vi "Fitting to battery model.vi"() -> ()   [LabVIEW 2013]
uses:
  <vilib>/Analysis/6fits.llb/Curve Fitting Criteria.ctl
  <vilib>/gmath/NumericalOptimization/Nonlinear Curve Fit LM bound.vi
  <vilib>/gmath/NI_Gmath.lvlib
  <vilib>/Analysis/NI_AALPro.lvlib
panel:
  out "residue":dbl
  out "number of function calls":i32
  out "Nyquist":cluster{dbl[], dbl[]}[](graph)
  out "p_best":dbl[](array[numeric])
  in  "p_init":dbl[](array[numeric])=[1e-06, 0.1, 0.1, 100.0, 1.0, 0.1, 0.1, 10.0, 0.1]
  out "f":dbl[](array[numeric])
  out "z":cdb[](array[numeric])
  in  "String":string="         1.000000E+4\t         4.126488E-2\t         2.967524E-1\n         8.912509E+3\t         4.158981E-2\t         2.604928E-1\n         7.943282E+3\t         4.199738E-2\t         2.277047E-1\n         7.079458E+3\t         4.250813E-2\t         1.979590E-1\n         6.309573E+3\t         4.314743E-2\t         1.708694E-1\n         5.623413E+3\t         4.394647E-2\t         1.460881E-1\n         5.011872E+3\t         4.494331E-2\t         1.233026E-1\n         4.466836E+3\t         4.618408E-2\t         1.022327E-1\n         3.981072E+3\t         4.772409E-2\t         8.262973E-2\n         3.548134E+3\t         4.962877E-2\t         6.427518E-2\n         3.162278E+3\t         5.197420E-2\t         4.698188E-2\n         2.818383E+3\t         5.484690E-2\t         3.059545E-2\n         2.511886E+3\t         5.834239E-2\t         1.499719E-2\n         2.238721E+3\t         6.256184E-2\t         1.075807E-4\n         1.995262E+3\t         6.760643E-2\t        -1.410996E-2\n         1.778279E+3\t         7.356869E-2\t        -2.764623E-2\n         1.584893E+3\t         8.052083E-2\t        -4.044574E-2\n         1.412538E+3\t         8.850068E-2\t        -5.241030E-2\n         1.258925E+3\t         9.749691E-2\t        -6.340858E-2\n         1.122018E+3\t         1.074364E-1\t        -7.329263E-2\n         1.000000E+3\t         1.181775E-1\t        -8.192073E-2\n         8.912509E+2\t         1.295128E-1\t        -8.918393E-2\n         7.943282E+2\t         1.411830E-1\t        -9.503155E-2\n         7.079458E+2\t         1.529012E-1\t        -9.948971E-2\n         6.309573E+2\t         1.643841E-1\t        -1.026685E-1\n         5.623413E+2\t         1.753820E-1\t        -1.047558E-1\n         5.011872E+2\t         1.857037E-1\t        -1.059995E-1\n         4.466836E+2\t         1.952307E-1\t        -1.066836E-1\n         3.981072E+2\t         2.039205E-1\t        -1.071023E-1\n         3.548134E+2\t         2.118007E-1\t        -1.075386E-1\n         3.162278E+2\t         2.189580E-1\t        -1.082484E-1\n         2.818383E+2\t         2.255252E-1\t        -1.094519E-1\n         2.511886E+2\t         2.316687E-1\t        -1.113294E-1\n         2.238721E+2\t         2.375799E-1\t        -1.140211E-1\n         1.995262E+2\t         2.434684E-1\t        -1.176284E-1\n         1.778279E+2\t         2.495579E-1\t        -1.222139E-1\n         1.584893E+2\t         2.560848E-1\t        -1.278009E-1\n         1.412538E+2\t         2.632954E-1\t        -1.343701E-1\n         1.258925E+2\t         2.714434E-1\t        -1.418538E-1\n         1.122018E+2\t         2.807835E-1\t        -1.501279E-1\n         1.000000E+2\t         2.915610E-1\t        -1.590041E-1\n         8.912509E+1\t         3.039956E-1\t        -1.682222E-1\n         7.943282E+1\t         3.182595E-1\t        -1.774476E-1\n         7.079458E+1\t         3.344495E-1\t        -1.862767E-1\n         6.309573E+1\t         3.525587E-1\t        -1.942534E-1\n         5.623413E+1\t         3.724514E-1\t        -2.009005E-1\n         5.011872E+1\t         3.938493E-1\t        -2.057633E-1\n         4.466836E+1\t         4.163370E-1\t        -2.084605E-1\n         3.981072E+1\t         4.393888E-1\t        -2.087338E-1\n         3.548134E+1\t         4.624172E-1\t        -2.064840E-1\n         3.162278E+1\t         4.848327E-1\t        -2.017841E-1\n         2.818383E+1\t         5.061048E-1\t        -1.948662E-1\n         2.511886E+1\t         5.258096E-1\t        -1.860854E-1\n         2.238721E+1\t         5.436572E-1\t        -1.758711E-1\n         1.995262E+1\t         5.594965E-1\t        -1.646750E-1\n         1.778279E+1\t         5.733007E-1\t        -1.529281E-1\n         1.584893E+1\t         5.851424E-1\t        -1.410095E-1\n         1.412538E+1\t         5.951632E-1\t        -1.292303E-1\n         1.258925E+1\t         6.035461E-1\t        -1.178289E-1\n         1.122018E+1\t         6.104913E-1\t        -1.069753E-1\n         1.000000E+1\t         6.161994E-1\t        -9.677938E-2\n         8.912509E+0\t         6.208601E-1\t        -8.730281E-2\n         7.943282E+0\t         6.246451E-1\t        -7.856953E-2\n         7.079458E+0\t         6.277055E-1\t        -7.057593E-2\n         6.309573E+0\t         6.301713E-1\t        -6.329917E-2\n         5.623413E+0\t         6.321524E-1\t        -5.670382E-2\n         5.011872E+0\t         6.337403E-1\t        -5.074691E-2\n         4.466836E+0\t         6.350109E-1\t        -4.538168E-2\n         3.981072E+0\t         6.360259E-1\t        -4.056024E-2\n         3.548134E+0\t         6.368360E-1\t        -3.623533E-2\n         3.162278E+0\t         6.374817E-1\t        -3.236156E-2\n         2.818383E+0\t         6.379962E-1\t        -2.889609E-2\n         2.511886E+0\t         6.384058E-1\t        -2.579904E-2\n         2.238721E+0\t         6.387317E-1\t        -2.303367E-2\n         1.995262E+0\t         6.389910E-1\t        -2.056638E-2\n         1.778279E+0\t         6.391972E-1\t        -1.836662E-2\n         1.584893E+0\t         6.393612E-1\t        -1.640677E-2\n         1.412538E+0\t         6.394915E-1\t        -1.466193E-2\n         1.258925E+0\t         6.395951E-1\t        -1.310973E-2\n         1.122018E+0\t         6.396774E-1\t        -1.173014E-2\n         1.000000E+0\t         6.397428E-1\t        -1.050524E-2\n         8.912509E-1\t         6.397948E-1\t        -9.419061E-3\n         7.943282E-1\t         6.398361E-1\t        -8.457384E-3\n         7.079458E-1\t         6.398690E-1\t        -7.607591E-3\n         6.309573E-1\t         6.398950E-1\t        -6.858504E-3\n         5.623413E-1\t         6.399158E-1\t        -6.200255E-3\n         5.011872E-1\t         6.399323E-1\t        -5.624158E-3\n         4.466836E-1\t         6.399454E-1\t        -5.122605E-3\n         3.981072E-1\t         6.399558E-1\t        -4.688965E-3\n         3.548134E-1\t         6.399642E-1\t        -4.317501E-3\n         3.162278E-1\t         6.399708E-1\t        -4.003298E-3\n         2.818383E-1\t         6.399761E-1\t        -3.742194E-3\n         2.511886E-1\t         6.399804E-1\t        -3.530732E-3\n         2.238721E-1\t         6.399839E-1\t        -3.366110E-3\n         1.995262E-1\t         6.399868E-1\t        -3.246146E-3\n         1.778279E-1\t         6.399892E-1\t        -3.169251E-3\n         1.584893E-1\t         6.399913E-1\t        -3.134406E-3\n         1.412538E-1\t         6.399931E-1\t        -3.141149E-3\n         1.258925E-1\t         6.399948E-1\t        -3.189571E-3\n         1.122018E-1\t         6.399964E-1\t        -3.280314E-3\n         1.000000E-1\t         6.399981E-1\t        -3.414583E-3\n         8.912509E-2\t         6.400000E-1\t        -3.594159E-3\n         7.943282E-2\t         6.400020E-1\t        -3.821424E-3\n         7.079458E-2\t         6.400044E-1\t        -4.099394E-3\n         6.309573E-2\t         6.400073E-1\t        -4.431755E-3\n         5.623413E-2\t         6.400108E-1\t        -4.822915E-3\n         5.011872E-2\t         6.400151E-1\t        -5.278063E-3\n         4.466836E-2\t         6.400205E-1\t        -5.803234E-3\n         3.981072E-2\t         6.400272E-1\t        -6.405390E-3\n         3.548134E-2\t         6.400355E-1\t        -7.092515E-3\n         3.162278E-2\t         6.400460E-1\t        -7.873714E-3\n         2.818383E-2\t         6.400592E-1\t        -8.759339E-3\n         2.511886E-2\t         6.400757E-1\t        -9.761117E-3\n         2.238721E-2\t         6.400965E-1\t        -1.089231E-2\n         1.995262E-2\t         6.401227E-1\t        -1.216788E-2\n         1.778279E-2\t         6.401557E-1\t        -1.360470E-2\n         1.584893E-2\t         6.401971E-1\t        -1.522173E-2\n         1.412538E-2\t         6.402493E-1\t        -1.704032E-2\n         1.258925E-2\t         6.403150E-1\t        -1.908441E-2\n         1.122018E-2\t         6.403977E-1\t        -2.138087E-2\n         1.000000E-2\t         6.405017E-1\t        -2.395982E-2\n         8.912509E-3\t         6.406325E-1\t        -2.685498E-2\n         7.943282E-3\t         6.407972E-1\t        -3.010405E-2\n         7.079458E-3\t         6.410044E-1\t        -3.374916E-2\n         6.309573E-3\t         6.412649E-1\t        -3.783725E-2\n         5.623413E-3\t         6.415925E-1\t        -4.242059E-2\n         5.011872E-3\t         6.420043E-1\t        -4.755720E-2\n         4.466836E-3\t         6.425218E-1\t        -5.331130E-2\n         3.981072E-3\t         6.431718E-1\t        -5.975371E-2\n         3.548134E-3\t         6.439876E-1\t        -6.696214E-2\n         3.162278E-3\t         6.450108E-1\t        -7.502134E-2\n         2.818383E-3\t         6.462931E-1\t        -8.402302E-2\n         2.511886E-3\t         6.478979E-1\t        -9.406533E-2\n         2.238721E-3\t         6.499034E-1\t        -1.052519E-1\n         1.995262E-3\t         6.524051E-1\t        -1.176902E-1\n         1.778279E-3\t         6.555185E-1\t        -1.314886E-1\n         1.584893E-3\t         6.593819E-1\t        -1.467524E-1\n         1.412538E-3\t         6.641590E-1\t        -1.635787E-1\n         1.258925E-3\t         6.700395E-1\t        -1.820481E-1\n         1.122018E-3\t         6.772392E-1\t        -2.022158E-1\n         1.000000E-3\t         6.859954E-1\t        -2.241001E-1\n"
  # "{ Ls, Rs, Rctc, Cdc, Cdlc, Rcta, Rda, Cda, Cdla }"
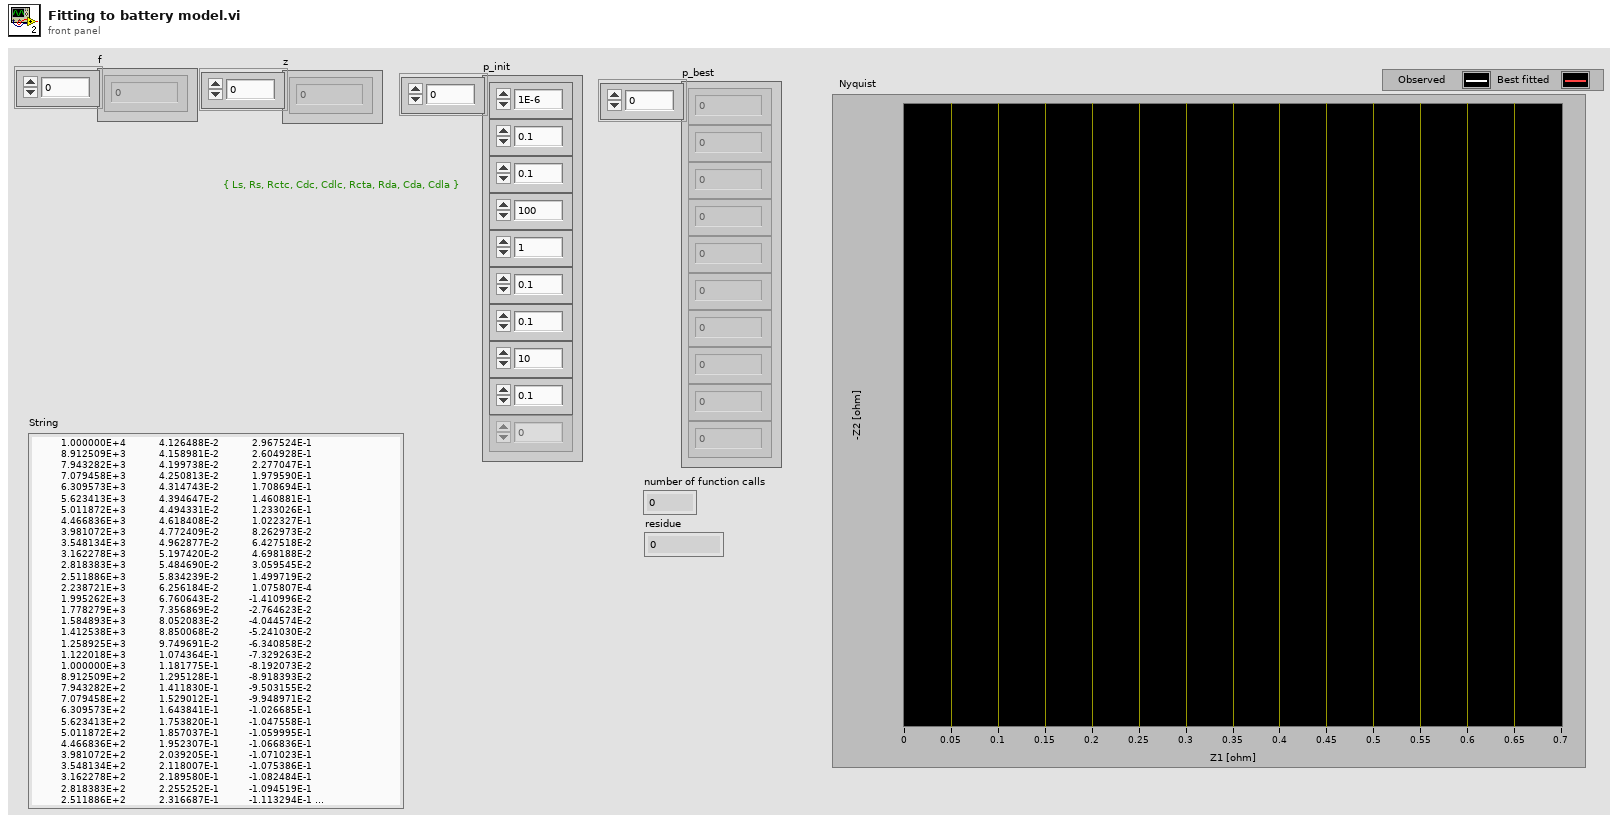
[diagram p1: front panel]
types:
  T1 = typedef "NI_AALPro.lvlib/Curve Fitting Criteria.ctl" = u16
  T2 = cluster{"parameter minimum":dbl[], "parameter maximum":dbl[]}
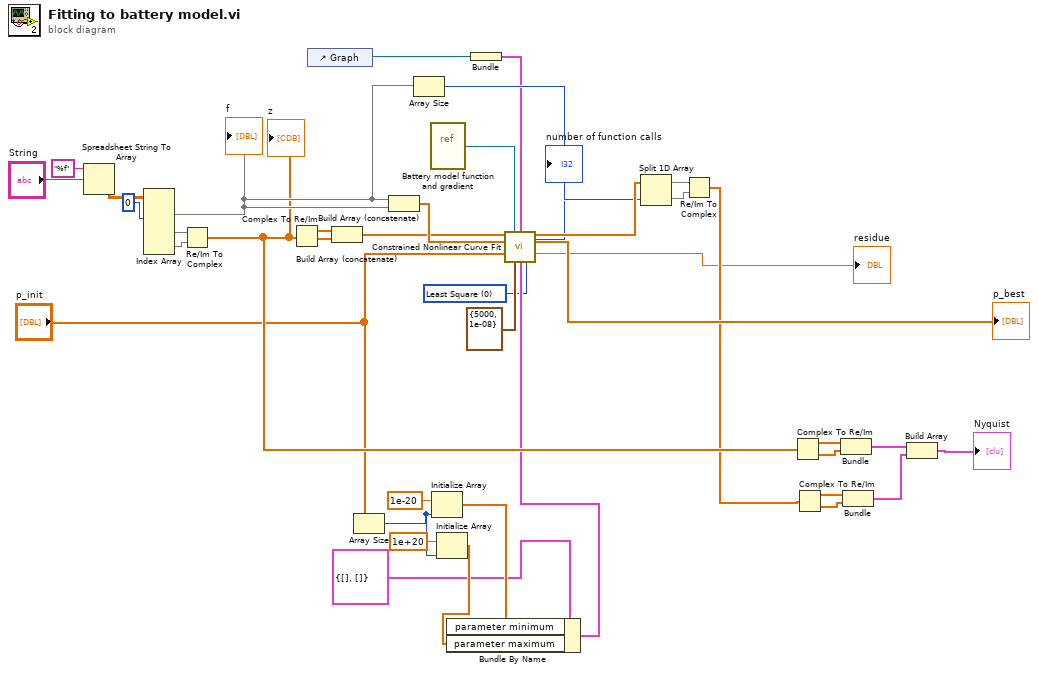
[diagram p0: block diagram]
diagram:
  w4 = T1 0 items=["Least Square", "Least Absolute Residual", "Bisquare"] ("method")
  n1 = Spreadsheet String To Array(format string="%f", spreadsheet string="String") -> (array=w38:dbl[][])  [unwired: 2 in]
  n2 = Index Array(array=w38, index (col) #1=0 ("disabled index (col)")) -> (element #1=w29:dbl[], element #2=w37:dbl[], element #3=w36:dbl[])  [unwired: 5 in]
  "f" <- w29
  n3 = Re/Im To Complex(1:w36, 2:w37) -> (0:w24:cdb[])
  "z" <- w24
  n4 = Complex To Re/Im(x + iy=w24) -> (x=w33:dbl[], y=w34:dbl[])
  n5 = control-ref of="Graph"() -> (w2:refnum<vi>)
  n6 = Build Array (concatenate)(w33, w34) -> (w6:dbl[])
  n7 = Array Size(array="p_init") -> (size(s)=w12:i32)
  n8 = Build Array (concatenate)(w29, w29) -> (w32:dbl[])
  n9 = Array Size(array=w29) -> (size(s)=w28:i32)
  n10 = vi-ref "Battery model function and gradient.vi"() -> (w31:refnum<vi>)
  n11 = Initialize Array(1e-20 ("element"), w12) -> (w11:dbl[])
  n12 = Initialize Array(1e+20 ("element"), w12) -> (w10:dbl[])
  n13 = Bundle By Name(cluster=T2 {"parameter minimum"=[], "parameter maximum"=[]} ("parameter bounds"), "parameter minimum"=w11, "parameter maximum"=w10) -> (w8:T2)
  n14 = Bundle("Graph"=w2) -> (w1:cluster{"Graph":refnum<vi>})  [unwired: 1 in]
  n15 = call-poly <vilib>:"Constrained Nonlinear Curve Fit.vi"("Y"=w6, "f(x,a)"=w31, "data"=w1, "X"=w32, "initial parameters"="p_init", "termination"=cluster{"max iteration":i32, "tolerance":dbl} {"max iteration"=5000, "tolerance"=1e-08}, "parameter bounds"=w8, "method"=w4) -> ("number of function calls"=→"number of function calls":i32, "best nonlinear fit"=w30:dbl[], "best fit parameters"=→"p_best":dbl[], "residue"=→"residue":dbl)  [unwired: 2 in, 2 out]
  n16 = Split 1D Array(array=w30, index=w28) -> (first subarray=w27:dbl[], second subarray=w26:dbl[])
  n17 = Re/Im To Complex(1:w26, 2:w27) -> (0:w19:cdb[])
  n18 = Complex To Re/Im(x + iy=w24) -> (x=w23:dbl[], y=w22:dbl[])
  n19 = Complex To Re/Im(x + iy=w19) -> (x=w20:dbl[], y=w21:dbl[])
  n20 = Bundle(w23, w22) -> (w18:cluster{dbl[], dbl[]})  [unwired: 1 in]
  n21 = Bundle(w20, w21) -> (w17:cluster{dbl[], dbl[]})  [unwired: 1 in]
  n22 = Build Array(w18, w17) -> (→"Nyquist":cluster{dbl[], dbl[]}[])
